vi "Ex1_Dig_Ang_Read.vi"() -> ()   [LabVIEW 2020]
uses:
  <vilib>/MakerHub/LINX/Public/Peripherals/Digital/Digital Read 1 Chan.vi
  <vilib>/MakerHub/LINX/Public/Peripherals/Analog/Analog Read 1 Chan.vi
  <vilib>/MakerHub/LINX/Public/Peripherals/Digital/Digital Read N Chans.vi
  <vilib>/MakerHub/LINX/Public/Peripherals/Analog/Analog Read N Chans.vi
  <vilib>/MakerHub/LINX/Private/Local IO/LinxDigitalRead.vi
  <vilib>/MakerHub/LINX/Public/Utilities/Check Channel.vi
  <vilib>/MakerHub/LINX/Private/Local IO/LinxAnalogRead.vi
  <vilib>/MakerHub/LINX/Public/Utilities/Open Serial.vi
  <vilib>/MakerHub/LINX/Private/Utilties/Generate Error.vi
  <vilib>/MakerHub/LINX/LMH-LINX.lvlib
panel:
  out "Analog2":dbl
  out "Digital2":bool
  out "Digital1":bool
  out "Analog1":dbl
  in  "stop":bool
  in  "Serial Port":refnum<visa-resource-name>="N/A"
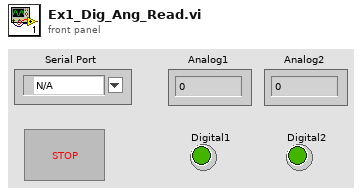
[diagram p1: front panel]
types:
  T1 = typedef "LMH-LINX.lvlib/LINX Ref.ctl" = cluster{"IO":T2, "Interface":T3, "LINX Device Config":T4}
  T2 = typedef "LMH-LINX.lvlib/Platform.ctl" = enum16{"Remote", "Local"}
  T3 = typedef "LMH-LINX.lvlib/Interface.ctl" = enum16{"Serial", "TCP"}
  T4 = typedef "LMH-LINX.lvlib/Device.lvlib/LINX Device Config.ctl" = cluster{"Interface":T3, "COM Port":refnum<visa-resource-name>, "TCP Configuration":T5, "Device Family":u8, "Device ID":u8, "Device Name":string, "TCP Ref":refnum<k5>, "Channels":T6}
  T5 = typedef "LMH-LINX.lvlib/Device.lvlib/TCP Config.ctl" = cluster{"IP Address":string, "Port":u16}
  T6 = typedef "LMH-LINX.lvlib/Channels.ctl" = cluster{"DI":u8[], "DO":u8[], "AI":u8[], "AO":u8[], "PWM":u8[], "QE":u8[], "UART":u8[], "I2C 2":u8[], "SPI":u8[], "CAN":u8[], "Servo":u8[], "AI Ref (V)":dbl, "AI Resolution (Bits)":u8, "AO Ref (V)":dbl, "AO Resolution (Bits)":u8}
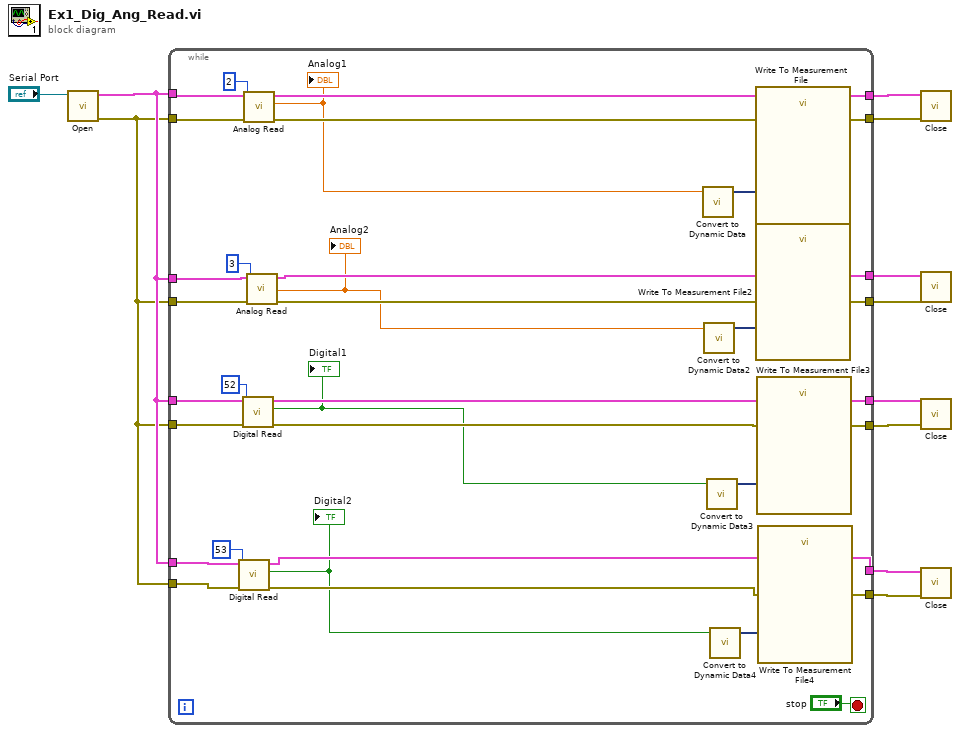
[diagram p0: block diagram]
diagram:
  n1 = call-poly <vilib>:"Open.vi"("Serial Port"="Serial Port") -> ("Error Out"=w7:errorcluster, "LINX Resource"=w8:T1)  [unwired: 8 in, 1 out]
  n2 = while {
    tunnel: w8 -> [w40]
    tunnel: w7 -> [w39]
    tunnel: [w38] -> w11
    tunnel: [w37] -> w10
    tunnel: w8 -> [w33]
    tunnel: w7 -> [w32]
    tunnel: w8 -> [w31]
    tunnel: w7 -> [w30]
    tunnel: w8 -> [w29]
    tunnel: w7 -> [w28]
    tunnel: [w25] -> w6
    tunnel: [w24] -> w5
    tunnel: [w23] -> w4
    tunnel: [w22] -> w3
    tunnel: [w21] -> w2
    tunnel: [w20] -> w1
    stop <- "stop" stop-if-true
    n3 = call-poly <vilib>:"Digital Read.vi"("Error In"=w28, "DI Channel"=u8 53, "LINX Resource"=w29) -> ("Error Out"=w20:errorcluster, "DI Value"=w12:bool, "LINX Resource"=w21:T1)  [unwired: 6 in]
    "Digital2" <- w12
    n4 = call-poly <vilib>:"Digital Read.vi"("Error In"=w30, "DI Channel"=u8 52, "LINX Resource"=w31) -> ("Error Out"=w22:errorcluster, "DI Value"=w14:bool, "LINX Resource"=w23:T1)  [unwired: 6 in]
    "Digital1" <- w14
    n5 = call-poly <vilib>:"Analog Read.vi"("Error In"=w39, "Analog Channel"=u8 2, "LINX Resource"=w40) -> ("Error Out"=w37:errorcluster, "Voltage"=w19:dbl, "LINX Resource"=w38:T1)  [unwired: 5 in, 1 out]
    "Analog1" <- w19
    n6 = call-poly <vilib>:"Analog Read.vi"("Error In"=w32, "Analog Channel"=u8 3, "LINX Resource"=w33) -> ("Error Out"=w24:errorcluster, "Voltage"=w16:dbl, "LINX Resource"=w25:T1)  [unwired: 5 in, 1 out]
    "Analog2" <- w16
    n7 = call "Convert to Dynamic Data"("Double"=w19) -> ("Dynamic Data Type"=w18:dynamicdata)  [unwired: 3 in]
    n8 = call "Convert to Dynamic Data2"("Double"=w16) -> ("Dynamic Data Type"=w17:dynamicdata)  [unwired: 3 in]
    n9 = call "Convert to Dynamic Data3"("Boolean"=w14) -> ("Dynamic Data Type"=w15:dynamicdata)  [unwired: 3 in]
    n10 = call "Convert to Dynamic Data4"("Boolean"=w12) -> ("Dynamic Data Type"=w13:dynamicdata)  [unwired: 3 in]
    n11 = call "Write To Measurement File"("Signals"=w18) -> ()  [unwired: 16 in, 3 out]
    n12 = call "Write To Measurement File2"("Signals"=w17) -> ()  [unwired: 16 in, 3 out]
    n13 = call "Write To Measurement File3"("Signals"=w15) -> ()  [unwired: 16 in, 3 out]
    n14 = call "Write To Measurement File4"("Signals"=w13) -> ()  [unwired: 16 in, 3 out]
  }
  n15 = call <vilib>:"Close.vi"("Error In"=w10, "LINX Resource"=w11) -> ()  [unwired: 9 in, 1 out]
  n16 = call <vilib>:"Close.vi"("Error In"=w5, "LINX Resource"=w6) -> ()  [unwired: 9 in, 1 out]
  n17 = call <vilib>:"Close.vi"("Error In"=w3, "LINX Resource"=w4) -> ()  [unwired: 9 in, 1 out]
  n18 = call <vilib>:"Close.vi"("Error In"=w1, "LINX Resource"=w2) -> ()  [unwired: 9 in, 1 out]
